vi "Example Main.vi"() -> ()   [LabVIEW 2014]
uses:
  vipm-to-nipm-package-converter/vipm-to-nipm-package-converter.lvlib
panel:
  out "Progress":u8(slide) scale=0.0..100.0
  in  "LabVIEW versions to support":string[](array[string])=["18.0"]
  out "Source VIPM packages with errors/warnings":path[](array[path])
  out "all errors/warnings":errorcluster[](array[cluster])
  out "Converted NIPM package filepaths":path[](array[path])
  in  "Source folder containing VIPM packages":path
  in  "Destination folder to place NIPM packages":path
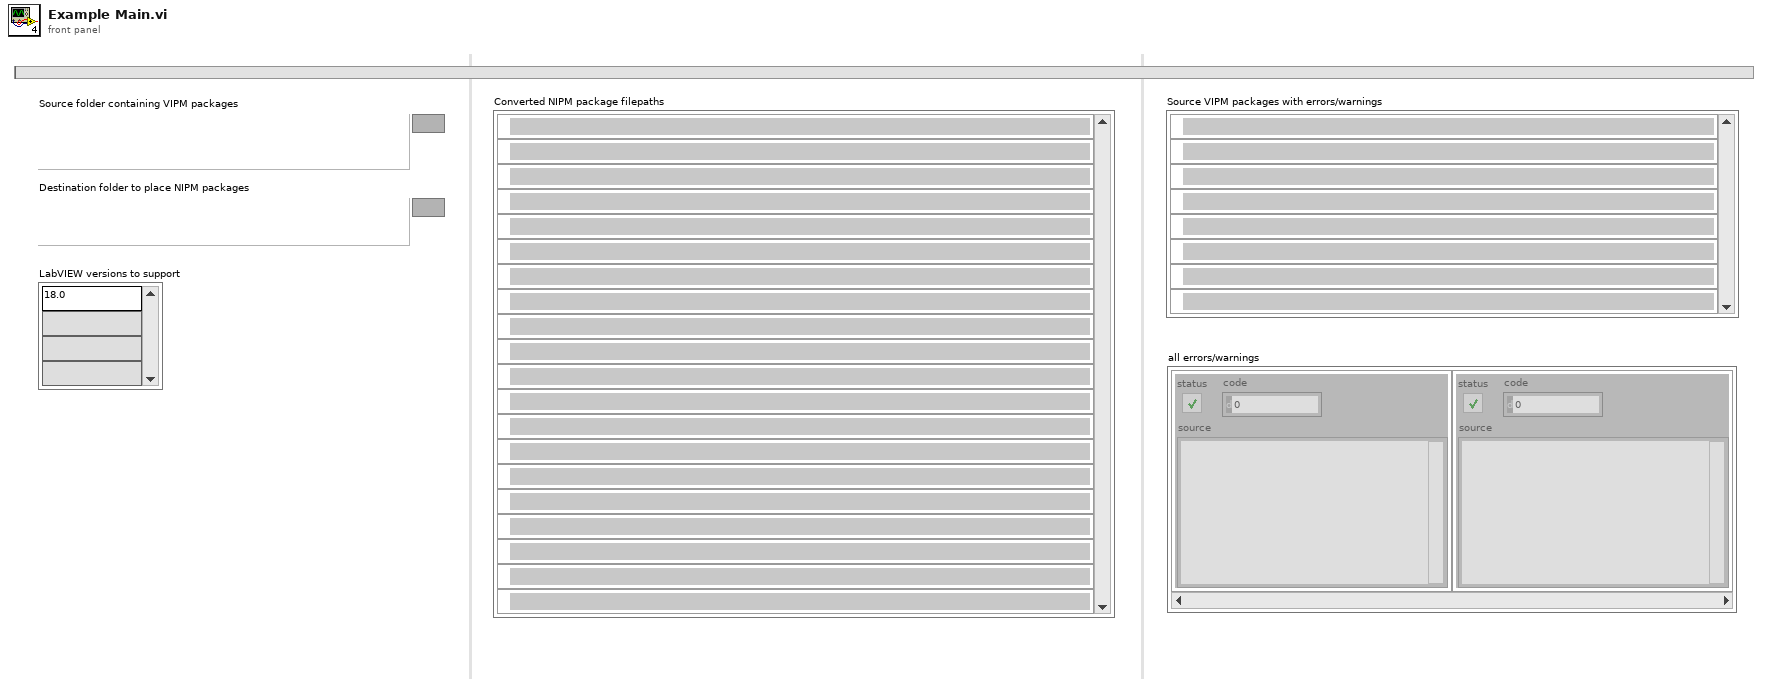
[diagram p1: front panel]
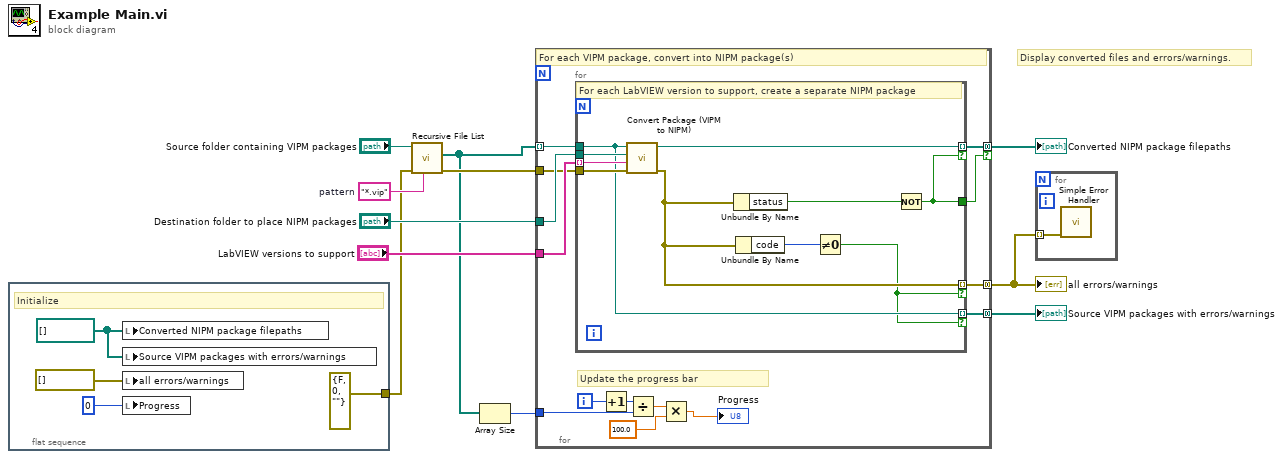
[diagram p0: block diagram]
diagram:
  w10 = "*.vip"  # pattern
  # "Display converted files and errors/warnings."
  n1 = flat-sequence {
    tunnel: [errorcluster {"status"=FALSE, "code"=0, "source"=""} ("error in (no error)")] -> w1
    frame #0 {
      w15 = path[] [] ("Converted NIPM package filepaths")
      # "Initialize"
      n2 = local write "Converted NIPM package filepaths"(w15) -> ()
      n3 = local write "Source VIPM packages with errors/warnings"(w15) -> ()
      n4 = local write "all errors/warnings"(errorcluster[] [] ("all errors/warnings")) -> ()
      n5 = local write "Progress"(u8 0 ("Progress")) -> ()
    }
  }
  n6 = call <vilib>:"Recursive File List.vi"("pattern"=w10, "error in (no error)"=w1, "Folder Path"="Source folder containing VIPM packages") -> ("error out"=w8:errorcluster, "All Files in Dir"=w4:path[])  [unwired: 4 in, 3 out]
  n7 = Array Size(array=w4) -> (size(s)=w3:i32)
  n8 = for {
    tunnel: "LabVIEW versions to support" -> [w29]
    tunnel: "Destination folder to place NIPM packages" -> [w28]
    tunnel: w4 -> [w26] mode=indexing
    tunnel: [w25] -> w6 mode=concatenating if=w23
    tunnel: [w24] -> w5 mode=concatenating
    tunnel: w3 -> [w20]
    tunnel: w8 -> [w27]
    tunnel: [w16] -> w2 mode=concatenating
    i -> [w22]
    # "Update the progress bar"
    # "For each VIPM package, convert into NIPM package(s)"
    n9 = for {
      tunnel: w29 -> [w39] mode=indexing
      tunnel: w28 -> [w38]
      tunnel: w26 -> [w33]
      tunnel: [w35] -> w25 mode=indexing if=w36
      tunnel: [w31] -> w24 mode=indexing if=w30
      tunnel: [w36] -> w23
      tunnel: w27 -> [w37]
      tunnel: [w33] -> w16 mode=indexing if=w30
      # "For each LabVIEW version to support, create a separate NIPM package"
      n10 = call "Convert Package (VIPM to NIPM).vi"("error in (no error)"=w37, "LabVIEW version"=w39, "Destination folder"=w38, "Source VIPM package (.vip)"=w33) -> ("error out"=w31:errorcluster, "Generated NIPM package (.nipkg)"=w35:path)  [unwired: 5 in, 1 out]
      n11 = Unbundle By Name(w31) -> ("status"=w34:bool)
      n12 = Unbundle By Name(w31) -> ("code"=w32:i32)
      n13 = Not Equal To 0?(x=w32) -> (x != 0?=w30:bool)
      n14 = Not(x=w34) -> (.not. x?=w36:bool)
    }
    n15 = Increment(x=w22) -> (x+1=w21:i32)
    n16 = Divide(x=w21, y=w20) -> (x/y=w19:dbl)
    n17 = Multiply(x=w19, y=100.0) -> (x*y=→"Progress":dbl)
  }
  "Converted NIPM package filepaths" <- w6
  "all errors/warnings" <- w5
  "Source VIPM packages with errors/warnings" <- w2
  n18 = for {
    tunnel: w5 -> [w40] mode=indexing
    n19 = call <vilib>:"Simple Error Handler.vi"("error in (no error)"=w40) -> ()  [unwired: 4 in, 5 out]
  }
